vi "Write.vi"(8 "error in":errorcluster, 9 "data":sgl[](array[numeric]), 10 "start index":i32=1, 11 "MicroDAQ.lvlib:DSP.lvclass":refnum<class "DSP.lvclass">) -> (0 "error out":errorcluster, 3 "MicroDAQ.lvlib:DSP.lvclass out":refnum<class "DSP.lvclass">)   [LabVIEW 2009, in "MicroDAQ.lvlib" / "DSP.lvclass"]
uses:
  <instrlib>/MicroDAQ/Channel/DSP/DSP.lvclass
  <instrlib>/MicroDAQ/Mlink library wraper/mlink.lvlib
  <instrlib>/MicroDAQ/Channel/Channel.lvclass
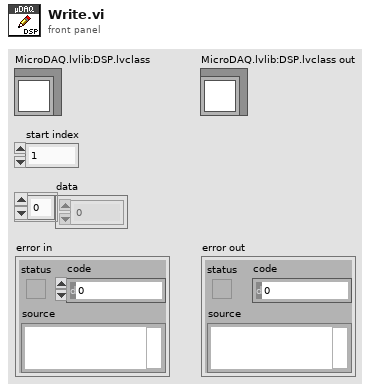
[diagram p1: front panel]
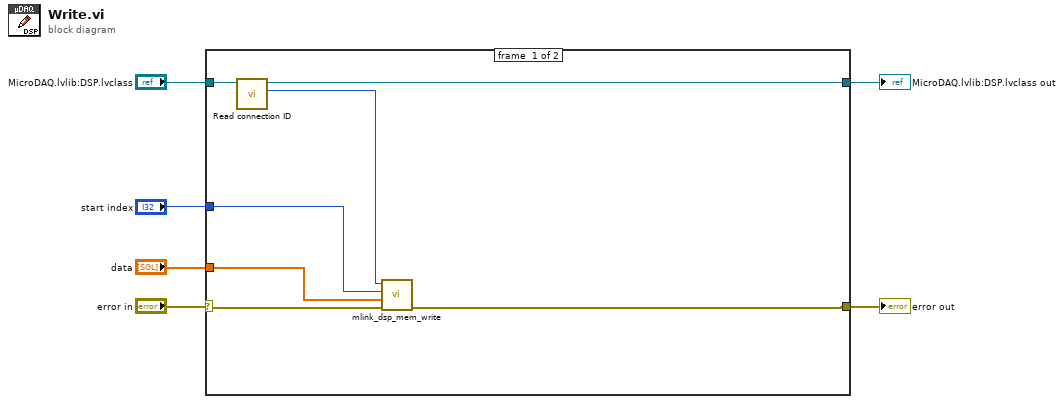
[diagram p0: block diagram]
diagram:
  n1 = case shown="No Error" "error in" {
    selector: "error in" -> [w10 w14]
    tunnel: "MicroDAQ.lvlib:DSP.lvclass" -> [w13 w15]
    tunnel: [w9 w14] -> w5
    tunnel: [w12 w15] -> w3
    tunnel: "data" -> [w8 _]
    tunnel: "start index" -> [w7 _]
    frame #0 {
      n2 = call <instrlib>:"Read connection ID.vi"("Task in"=w13) -> ("connection ID"=w11:i32, "Task out"=w12:refnum<class "DSP.lvclass">)  [unwired: 9 in]
      n3 = call <instrlib>:"mlink_dsp_mem_write.vi"("error in (no error)"=w10, "data"=w8, "start index"=w7, "connection ID"=w11) -> ("error put"=w9:errorcluster)  [unwired: 6 in, 1 out]
    }
    frame #1 {
    }
  }
  "error out" <- w5
  "MicroDAQ.lvlib:DSP.lvclass out" <- w3
